vi "Get Fault List.vi"(8 "error in (no error)":errorcluster) -> (0 "error out":errorcluster, 2 "fault list":T1[](array[typedef]) {"level" items=["Minor Fault", "Major Fault", "Unrecoverable Fault"]})   [LabVIEW 2020]
doc: "Returns a list of active faults."
uses:
  <vilib>/NIScanEngine/faults/Fault.ctl
  <resource>/objmgr/ni.var.rc
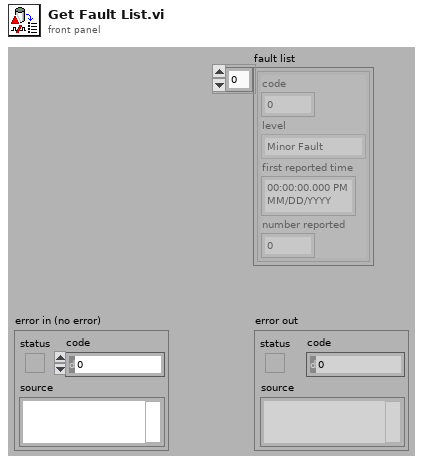
[diagram p1: front panel]
types:
  T1 = typedef "Fault.ctl" = cluster{"code":i32, "level":i32, "first reported time":timestamp, "number reported":u32}
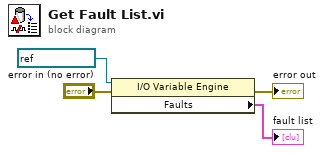
[diagram p0: block diagram]
diagram:
  n1 = property class="I/O Variable Engine"(reference=refnum<k21> "ni.var.io:/" ("reference out"), error in="error in (no error)") -> (error out=→"error out":errorcluster, "Faults"=→"fault list":T1[])  [unwired: 1 out]
